vi "SwerveModuleState_CompareTo.vi"(9 "other SWERVE_DRIVE_MODULE_STATE":T1={"Speed"=0.0, "Angle"={"VALUE"=0.0, "COS"=1.0, "SIN"=0.0}} {"Angle"."SIN" format="%13.4f"; "Angle"."COS" format="%13.4f"; "Angle"."VALUE" format="%13.4f"}, 11 "in SWERVE_DRIVE_MODULE_STATE":T1={"Speed"=0.0, "Angle"={"VALUE"=0.0, "COS"=1.0, "SIN"=0.0}} {"Angle"."SIN" format="%13.4f"; "Angle"."COS" format="%13.4f"; "Angle"."VALUE" format="%13.4f"}) -> (3 "Compare":i32)   [LabVIEW 2019, in "Trajectory_Library.lvlib"]
doc: "Compares two swerve module states. One swerve module is \"greater\" than the other if its speed is higher than the other.\n\nParmeters:\n - this Module State\n - other Module State - The other swerve module.\n\nReturns:\n - compare - comparison result where\n 1 if this is greater, \n 0 if both are equal, \n -1 if other is greater."
uses:
  Trajectory_Library.lvlib
  TypeDef/SWERVE_DRIVE_MODULE_STATE.ctl
  TypeDef/ROTATION2D.ctl
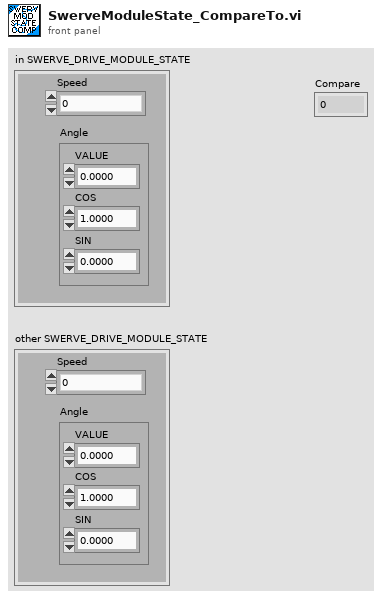
[diagram p1: front panel]
types:
  T1 = typedef "Trajectory_Library.lvlib/SWERVE_DRIVE_MODULE_STATE.ctl" = cluster{"Speed":dbl, "Angle":T2}
  T2 = typedef "Trajectory_Library.lvlib/ROTATION2D.ctl" = cluster{"VALUE":dbl, "COS":dbl, "SIN":dbl}
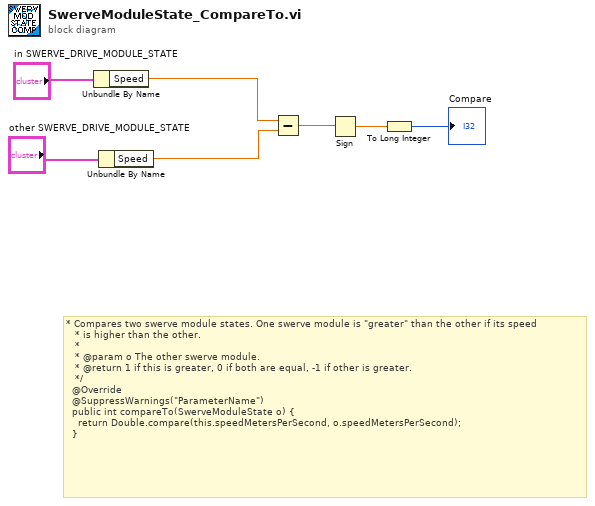
[diagram p0: block diagram]
diagram:
  # "* Compares two swerve module states. One swerve module is \"greater\" than the other if its speed\n   * is higher than the other.\n   *\n   * @param o The other swerve module.\n   * @return 1 if this is greater, 0 if both are equal, -1 if other is greater.\n   */\n  @Override\n  @SuppressWarnings(\"ParameterName\")\n  public int compareTo(SwerveModuleState o) {\n    return Double.compare(this.speedMetersPerSecond, o.speedMetersPerSecond);\n  }"
  n1 = Unbundle By Name("in SWERVE_DRIVE_MODULE_STATE") -> ("Speed"=w5:dbl)
  n2 = Unbundle By Name("other SWERVE_DRIVE_MODULE_STATE") -> ("Speed"=w4:dbl)
  n3 = Subtract(x=w5, y=w4) -> (x-y=w3:dbl)
  n4 = Sign(1:w3) -> (0:w2:dbl)
  n5 = To Long Integer(number=w2) -> (32bit integer=→"Compare":i32)
